vi "Queues - DeInit.vi"(8 "error in (no error)":errorcluster, 11 "Queues":T1) -> (0 "error out":errorcluster)   [LabVIEW 2017]
doc: "Initialize all queues in application"
uses:
  Controls/Queues.ctl
  Controller/Controls/Controller CMD.ctl
  Configuration/Controls/Config CMD.ctl
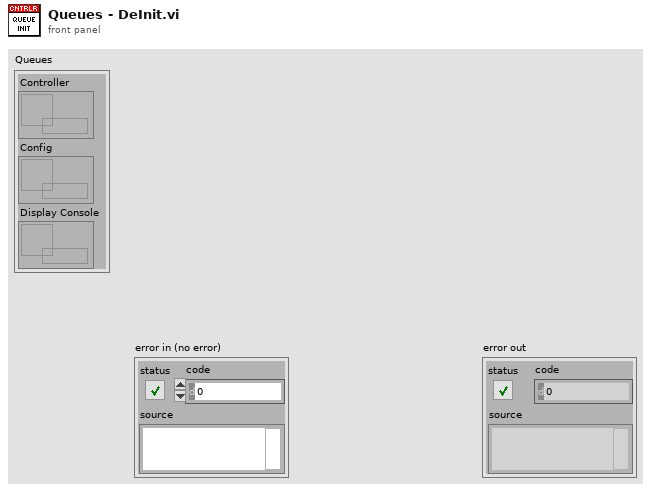
[diagram p1: front panel]
types:
  T1 = typedef "Queues.ctl" = cluster{"Controller":refnum<queue>, "Config":refnum<queue>, "Display Console":refnum<queue>}
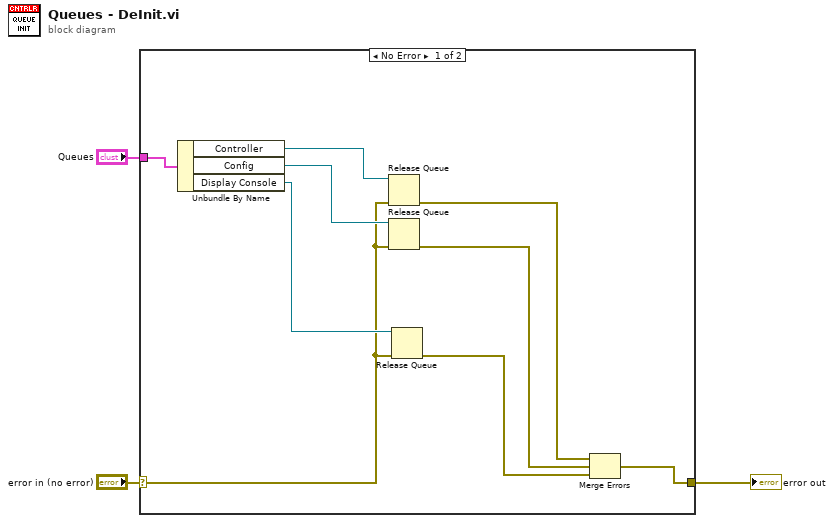
[diagram p0: block diagram]
diagram:
  n1 = case shown="No Error" "error in (no error)" {
    selector: "error in (no error)" -> [w5 w13]
    tunnel: [w7 w13] -> w2
    tunnel: "Queues" -> [w12 _]
    frame No Error {
      n2 = Unbundle By Name(w12) -> ("Controller"=w11:refnum<queue>, "Config"=w10:refnum<queue>, "Display Console"=w6:refnum<queue>)
      n3 = Release Queue(queue=w11, error in (no error)=w5) -> (error out=w9:errorcluster)  [unwired: 1 in, 2 out]
      n4 = Release Queue(queue=w10, error in (no error)=w5) -> (error out=w8:errorcluster)  [unwired: 1 in, 2 out]
      n5 = Release Queue(queue=w6, error in (no error)=w5) -> (error out=w4:errorcluster)  [unwired: 1 in, 2 out]
      n6 = Merge Errors(w9, w8, w4) -> (w7:errorcluster)
    }
    frame Error {
    }
  }
  "error out" <- w2
